vi "Set initialize.vi"(8 "error in (no error)":errorcluster, 11 "VISA resource name":refnum<visa-resource-name>="COM4") -> (0 "error out":errorcluster, 2 "Initialize Output":string, 3 "VISA resource name out":refnum<visa-resource-name>)   [LabVIEW 2017]
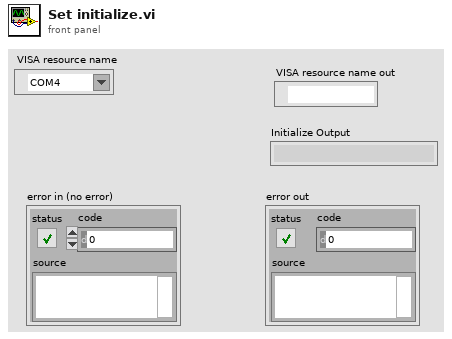
[diagram p1: front panel]
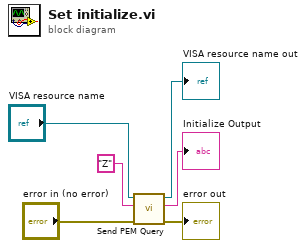
[diagram p0: block diagram]
diagram:
  n1 = call "Send PEM Query.vi"("error in (no error)"="error in (no error)", "query string"="Z", "VISA resource name"="VISA resource name") -> ("error out"=→"error out":errorcluster, "query output"=→"Initialize Output":string, "VISA resource name out"=→"VISA resource name out":refnum<visa-resource-name>)  [unwired: 5 in, 1 out]
